vi "chopdata2.vi"(8 "velo":dbl[][](array[numeric]), 9 "pos":dbl[](array[numeric])) -> (1 "slam_pos":dbl[](array[numeric]))   [LabVIEW 2012]
uses:
  G_SEN.vi
  <vilib>/Analysis/baseanly.llb/Real A x B.vi
  <vilib>/Analysis/7linalg.llb/Real SVD Decomposition.vi
  <vilib>/Analysis/Matrix/Numeric/Multiply/Multiply - RM,RM.vi
  <vilib>/Analysis/baseanly.llb/A x Vector.vi
  <vilib>/Analysis/Matrix/Numeric/Conversions/Matrix To Array - RM.vi
  <vilib>/Analysis/NI_AALBase.lvlib
  <vilib>/Analysis/NI_AALPro.lvlib
  <vilib>/Analysis/Matrix/NI_Matrix.lvlib
panel:
  out "Array 2":dbl[][](array[numeric])
  out "Array":dbl[](array[numeric])
  out "thresh":dbl
  out "iter":i32
  in  "y 2":dbl
  in  "graph":bool
  out "error":dbl
  out "R'":dbl[][](array[numeric])
  out "y'":dbl
  out "x'":dbl
  out "mindata":dbl[][](array[numeric])
  out "keydata":dbl[][](array[numeric])
  out "zero_80_240":i32[][](array[numeric])
  out "time":u32
  out "x":dbl[](array[numeric])
  out "y":dbl[](array[numeric])
  out "XY Graph":cluster{"Y":dbl[], "Y":dbl[]}[](graph)
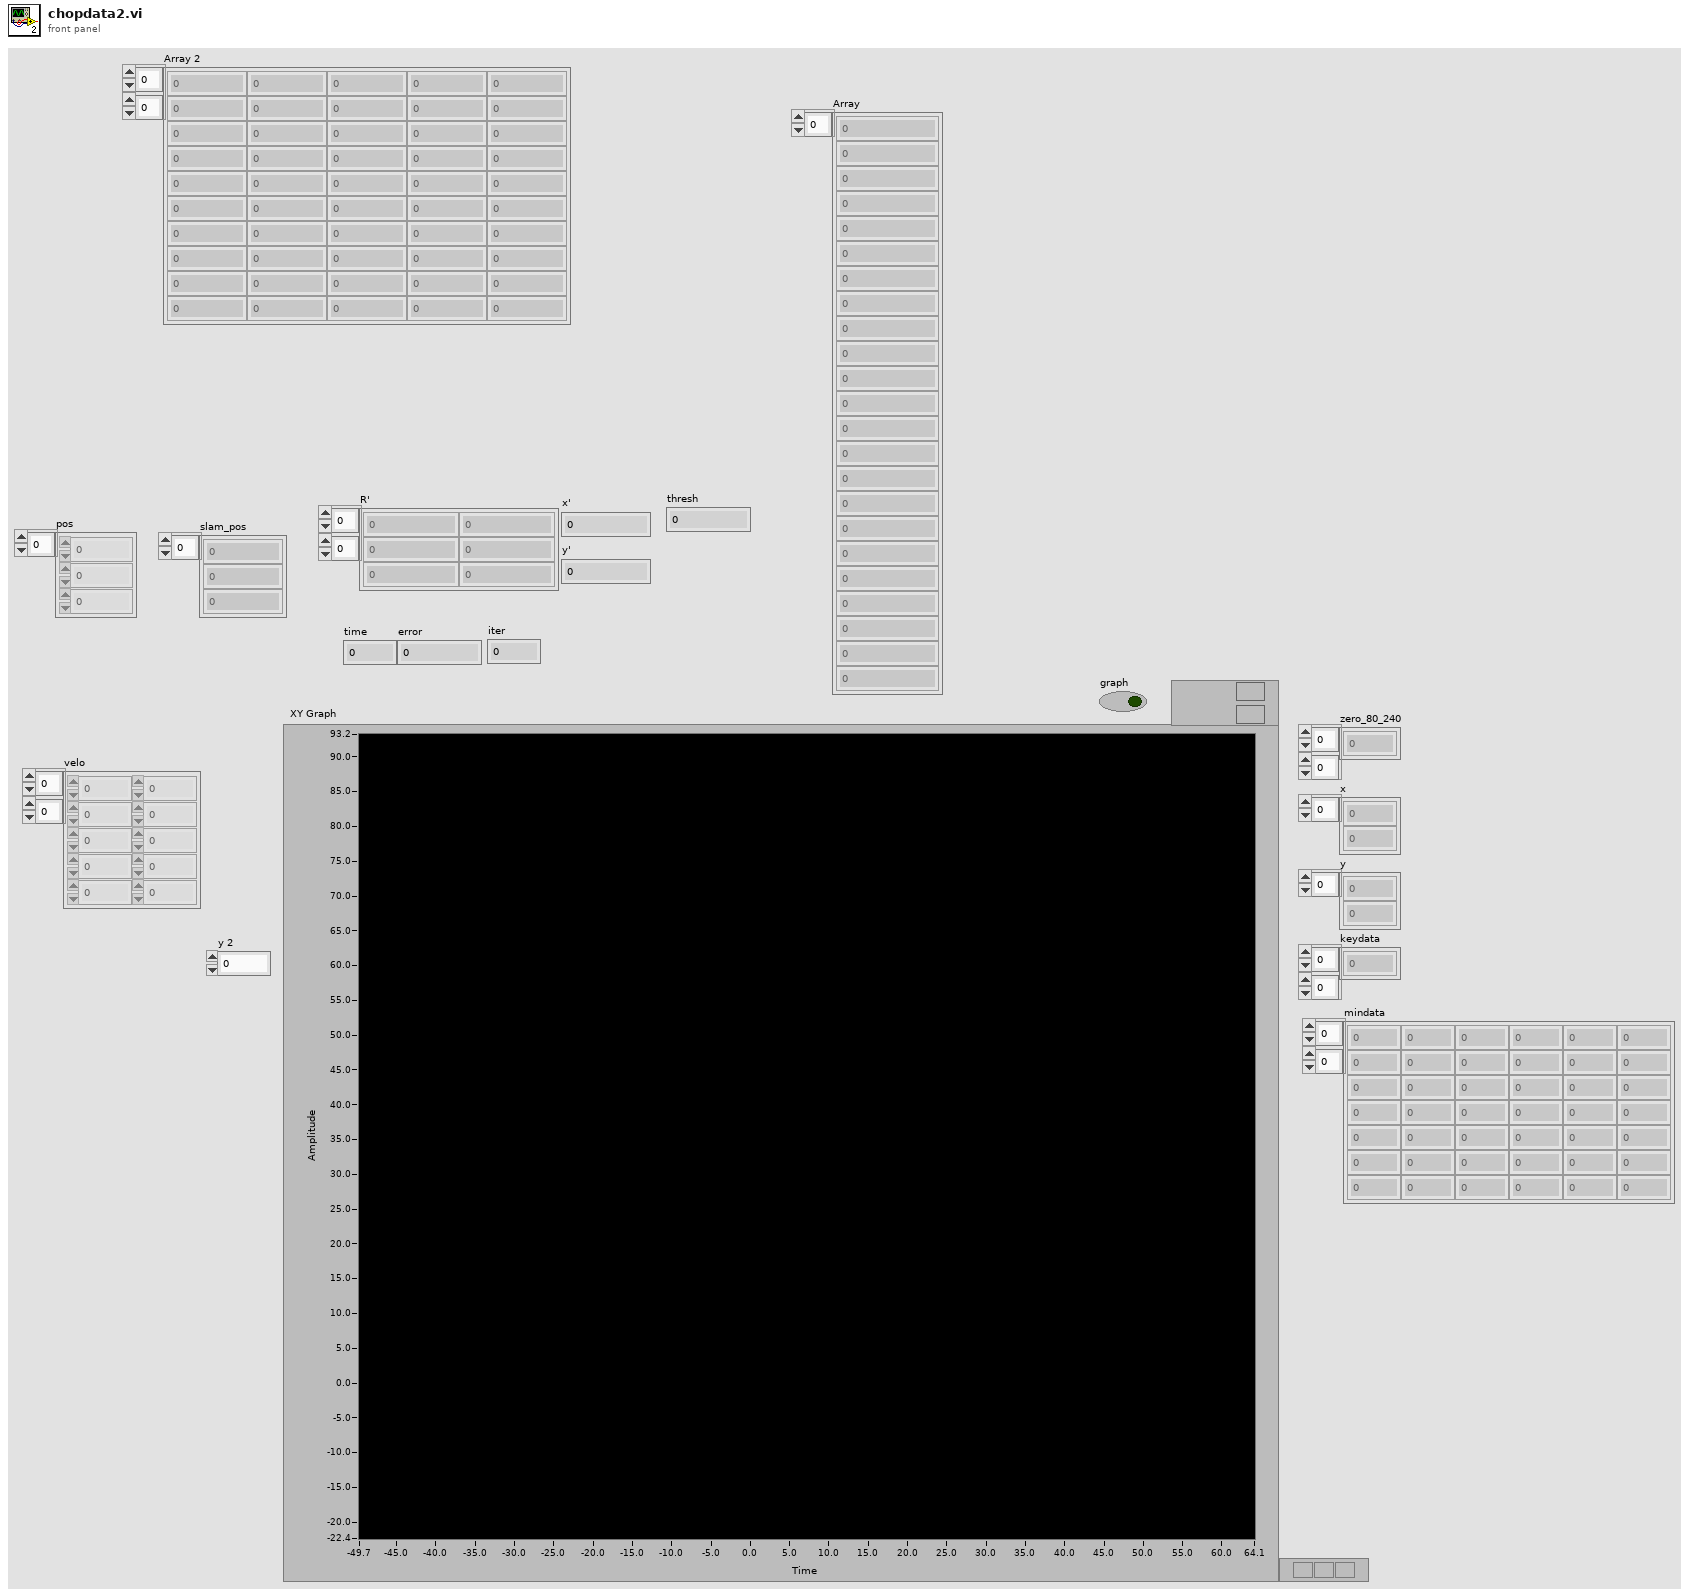
[diagram p1: front panel]
types:
  T1 = cluster{bool, "element":dbl, "element":dbl, "element":dbl}[]
  T2 = cluster{"element":bool, "element":dbl, "element":dbl, "element":dbl}[]
  T3 = typedef "NI_Matrix.lvlib/RealMatrix.ctl" = dbl[][]
  T4 = cluster{"Real Matrix Element":bool, "Real Matrix Element":dbl, "Real Matrix Element":dbl}[]
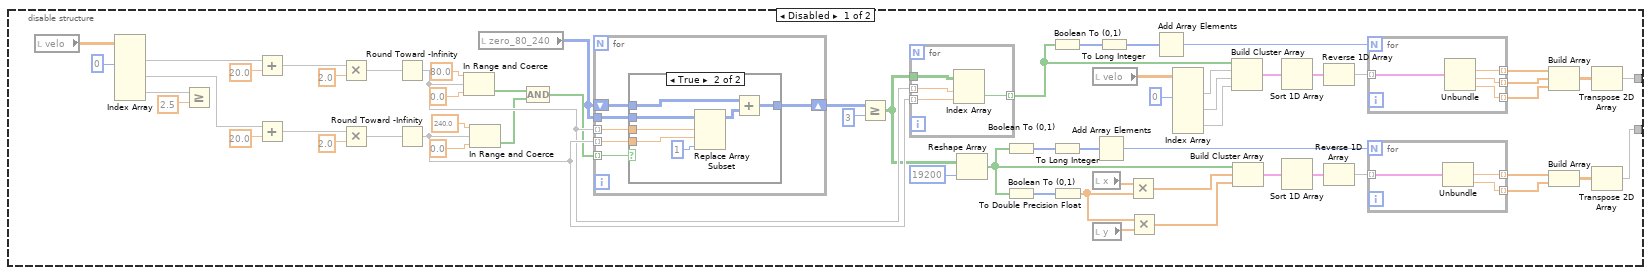
[diagram p3: hidden frame]
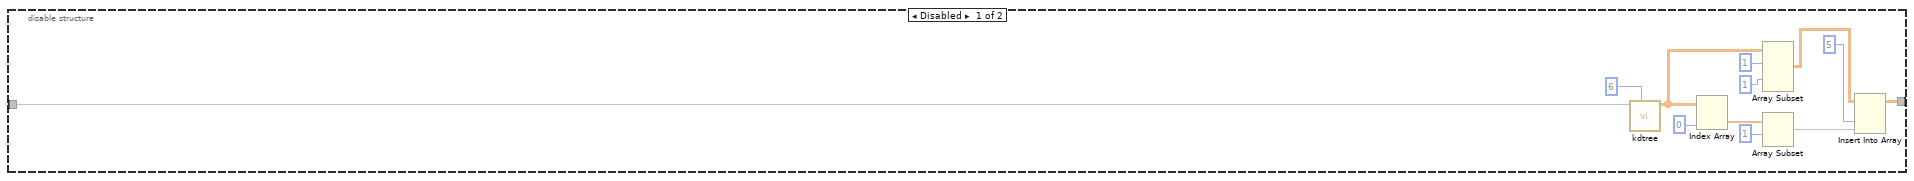
[diagram p5: hidden frame]
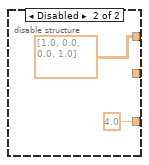
[diagram p7: hidden frame]
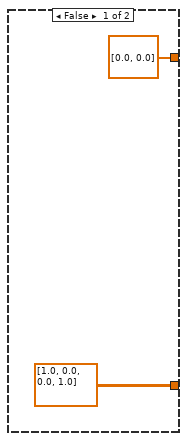
[diagram p9: hidden frame]
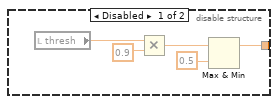
[diagram p10: hidden frame]
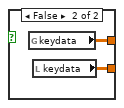
[diagram p12: hidden frame]
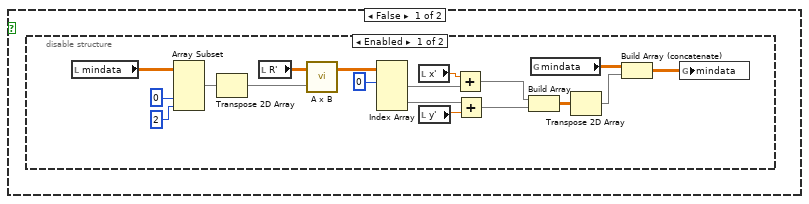
[diagram p13: hidden frame]
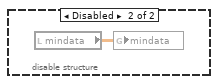
[diagram p15: hidden frame]
diagram:
  n1 = flat-sequence {
    tunnel: [w37] -> w6
    tunnel: w6 -> [w40]
    tunnel: [w40] -> w1
    tunnel: w1 -> [w255]
    tunnel: [w255] -> w5
    tunnel: w5 -> [w265]
    tunnel: [w265] -> w4
    tunnel: w4 -> [w295]
    tunnel: [w295] -> w3
    tunnel: w3 -> [w518]
    tunnel: [w518] -> w2
    tunnel: w2 -> [w520]
    frame #0 {
      n2 = First Call?() -> (First Call?: T/F=w7:bool)
      n3 = case shown="True" w7 {
        frame False {
        }
        frame True {
          n4 = Initialize Array(0, 80 ("dimension size"), 240 ("dimension size")) -> (→"zero_80_240":i32[][])
          n5 = for {
            N: 80 -> [_]
            tunnel: -19.75 -> [w27]
            tunnel: [w24] -> w12 mode=indexing
            tunnel: [w23] -> w17 mode=indexing
            i -> [w26]
            n6 = To Double Precision Float(number=w26) -> (double precision float=w22:dbl)
            n7 = Multiply(x=w22, y=0.5) -> (x*y=w20:dbl)
            n8 = Add(x=w27, y=w20) -> (x+y=w25:dbl)
            n9 = for {
              N: 240 -> [_]
              tunnel: -19.75 -> [w36]
              tunnel: [w34] -> w23 mode=indexing
              tunnel: w25 -> [w33]
              tunnel: [w33] -> w24 mode=indexing
              i -> [w35]
              n10 = To Double Precision Float(number=w35) -> (double precision float=w32:dbl)
              n11 = Multiply(x=w32, y=0.5) -> (x*y=w30:dbl)
              n12 = Add(x=w36, y=w30) -> (x+y=w34:dbl)
            }
          }
          n13 = Reshape Array(w17, 19200 ("dimension size")) -> (→"y":dbl[])
          n14 = Reshape Array(w12, 19200 ("dimension size")) -> (→"x":dbl[])
        }
      }
    }
    frame #1 {
      n15 = Tick Count (ms)() -> (millisecond timer value=w37:u32)
    }
    frame #2 {
      n16 = disable-structure shown="Enabled" {
        disable-tunnel: [w44 w129] -> w39
        disable-tunnel: [w43 w128] -> w38
        frame Disabled {
          n17 = local read "velo"() -> (w50:dbl[][])
          n18 = Index Array(array=w50, index (col) #1=0 ("disabled index (col)")) -> (element #1=w79:dbl[], element #2=w78:dbl[], element #3=w42:dbl[])  [unwired: 5 in]
          n19 = Greater Or Equal?(x=w42, y=2.5) -> ()  [unwired: 1 out]
          n20 = Add(x=w79, y=20.0) -> (x+y=w75:dbl[])
          n21 = Add(x=w78, y=20.0) -> (x+y=w71:dbl[])
          n22 = Multiply(x=w75, y=2.0) -> (x*y=w74:dbl[])
          n23 = Multiply(x=w71, y=2.0) -> (x*y=w70:dbl[])
          n24 = Round Toward -Infinity(1:w74) -> (0:w92:dbl[])
          n25 = Round Toward -Infinity(1:w70) -> (0:w93:dbl[])
          n26 = In Range and Coerce(upper limit=80.0, x=w92, lower limit=0.0) -> (In Range?=w87:bool[])  [unwired: 1 out]
          n27 = In Range and Coerce(upper limit=240.0, x=w93, lower limit=0.0) -> (In Range?=w88:bool[])  [unwired: 1 out]
          n28 = local read "zero_80_240"() -> (w54:i32[][])
          n29 = Compound Arithmetic op=AND(w87, w88) -> (w89:bool[])
          n30 = for {
            shift-right: [w117] -> w91
            shift-left: w54 -> [w118]
            tunnel: w89 -> [w119] mode=indexing
            tunnel: w54 -> [w116]
            tunnel: w92 -> [w115] mode=indexing
            tunnel: w93 -> [w114] mode=indexing
            n31 = case shown="True" w119 {
              tunnel: w118 -> [w120 w123]
              tunnel: [w120 w121] -> w117
              tunnel: w116 -> [_ w127]
              tunnel: w115 -> [_ w126]
              tunnel: w114 -> [_ w125]
              frame False {
              }
              frame True {
                n32 = Replace Array Subset(array=w127, new element=1 ("new element/subarray"), index (row)=w126, index (col)=w125) -> (w122:i32[][])
                n33 = Add(x=w123, y=w122) -> (x+y=w121:i32[][])
              }
            }
          }
          n34 = Greater Or Equal?(x=w91, y=3) -> (x >= y?=w63:bool[][])
          n35 = for {
            tunnel: w63 -> [w113]
            tunnel: w92 -> [w112] mode=indexing
            tunnel: w93 -> [w111] mode=indexing
            tunnel: [w110] -> w96 mode=indexing
            n36 = Index Array(array=w113, index (row)=w112, index (col)=w111) -> (element=w110:bool)
          }
          n37 = Reshape Array(w63, 19200 ("dimension size")) -> (w57:bool[])
          n38 = Boolean To (0,1)(Boolean=w57) -> (0, 1=w59:i16[])
          n39 = Boolean To (0,1)(Boolean=w57) -> (0, 1=w68:i16[])
          n40 = Boolean To (0,1)(Boolean=w96) -> (0, 1=w97:i16[])
          n41 = To Long Integer(number=w59) -> (32bit integer=w58:i32[])
          n42 = To Double Precision Float(number=w68) -> (double precision float=w62:dbl[])
          n43 = local read "velo"() -> (w49:dbl[][])
          n44 = local read "x"() -> (w66:dbl[])
          n45 = local read "y"() -> (w67:dbl[])
          n46 = Add Array Elements(numeric array=w58) -> (sum=w56:i32)
          n47 = To Long Integer(number=w97) -> (32bit integer=w98:i32[])
          n48 = Multiply(x=w66, y=w62) -> (x*y=w65:dbl[])
          n49 = Multiply(x=w62, y=w67) -> (x*y=w64:dbl[])
          n50 = Add Array Elements(numeric array=w98) -> (sum=w99:i32)
          n51 = Index Array(array=w49, index (col) #1=0 ("disabled index (col)")) -> (element #1=w47:dbl[], element #2=w46:dbl[], element #3=w45:dbl[])  [unwired: 5 in]
          n52 = Build Cluster Array(w96, w47, w46, w45) -> (w94:T1)
          n53 = Build Cluster Array(w57, w65, w64) -> (w60:cluster{bool, dbl, dbl}[])
          n54 = Sort 1D Array(array=w94) -> (sorted array=w95:T1)
          n55 = Sort 1D Array(array=w60) -> (sorted array=w61:cluster{bool, dbl, dbl}[])
          n56 = Reverse 1D Array(array=w95) -> (reversed array=w100:T1)
          n57 = Reverse 1D Array(array=w61) -> (reversed array=w55:cluster{bool, dbl, dbl}[])
          n58 = for {
            N: w99 -> [_]
            tunnel: w100 -> [w109] mode=indexing
            tunnel: [w108] -> w77 mode=indexing
            tunnel: [w107] -> w76 mode=indexing
            tunnel: [w106] -> w101 mode=indexing
            n59 = Unbundle(w109) -> ("element"=w108:dbl, "element"=w107:dbl, "element"=w106:dbl)  [unwired: 1 out]
          }
          n60 = for {
            N: w56 -> [_]
            tunnel: w55 -> [w105] mode=indexing
            tunnel: [w104] -> w53 mode=indexing
            tunnel: [w103] -> w52 mode=indexing
            n61 = Unbundle(w105) -> (w104:dbl, w103:dbl)  [unwired: 1 out]
          }
          n62 = Build Array(w77, w76, w101) -> (w102:dbl[][])
          n63 = Build Array(w53, w52) -> (w51:dbl[][])
          n64 = Transpose 2D Array(2D array=w102) -> (transposed array=w44:dbl[][])
          n65 = Transpose 2D Array(2D array=w51) -> (transposed array=w43:dbl[][])
        }
        frame Enabled {
          n66 = local read "velo"() -> (w130:dbl[][])
          n67 = flat-sequence {
            tunnel: w130 -> [w158]
            tunnel: [w133] -> w129
            frame #0 {
              n68 = Index Array(array=w158, index (col) #1=0 ("disabled index (col)")) -> (element #1=w157:dbl[], element #2=w152:dbl[], element #3=w132:dbl[])  [unwired: 5 in]
              n69 = Greater?(x=w132, y=0) -> ()  [unwired: 1 out]
              n70 = In Range and Coerce(upper limit=40.0, x=w152, lower limit=0.0) -> (In Range?=w150:bool[])  [unwired: 1 out]
              n71 = In Range and Coerce(upper limit=40.0, x=w157, lower limit=-40.0) -> (In Range?=w151:bool[])  [unwired: 1 out]
              n72 = local read "velo"() -> (w139:dbl[][])
              n73 = Compound Arithmetic op=AND(w151, w150) -> (w134:bool[])
              n74 = Index Array(array=w139, index (col) #1=0 ("disabled index (col)")) -> (element #1=w137:dbl[], element #2=w136:dbl[], element #3=w135:dbl[])  [unwired: 5 in]
              n75 = Boolean To (0,1)(Boolean=w134) -> (0, 1=w144:i16[])
              n76 = Build Cluster Array(w134, w137, w136, w135) -> (w142:T2)
              n77 = To Long Integer(number=w144) -> (32bit integer=w145:i32[])
              n78 = Sort 1D Array(array=w142) -> (sorted array=w143:T2)
              n79 = Add Array Elements(numeric array=w145) -> (sum=w146:i32)
              n80 = Reverse 1D Array(array=w143) -> (reversed array=w147:T2)
              n81 = for {
                N: w146 -> [_]
                tunnel: w147 -> [w163] mode=indexing
                tunnel: [w162] -> w141 mode=indexing
                tunnel: [w161] -> w140 mode=indexing
                tunnel: [w160] -> w148 mode=indexing
                n82 = Unbundle(w163) -> ("element"=w162:dbl, "element"=w161:dbl, "element"=w160:dbl)  [unwired: 1 out]
              }
              n83 = Build Array(w141, w140, w148) -> (w149:dbl[][])
              n84 = Transpose 2D Array(2D array=w149) -> (transposed array=w133:dbl[][])
            }
          }
          n85 = disable-structure shown="Enabled" {
            disable-tunnel: w129 -> [w175 w183]
            disable-tunnel: [w167 w176] -> w128
            frame Disabled {
              n86 = call "kdtree.vi"("depth_max"=6, "in"=w175) -> ("out"=w171:dbl[][])  [unwired: 8 in, 1 out]
              n87 = Index Array(array=w171, index (col)=0 ("disabled index (col)")) -> (element=w166:dbl[])  [unwired: 1 in]
              n88 = Array Subset(array=w171, index (row)=1 ("index"), index (col)=1 ("index")) -> (w169:dbl[][])  [unwired: 2 in]
              n89 = Array Subset(array=w166, index=1) -> (w164:dbl[])  [unwired: 1 in]
              n90 = Insert Into Array(array=w169, index (col)=5 ("disabled index (col)"), new element=w164) -> (w167:dbl[][])  [unwired: 1 in]
            }
            frame Enabled {
              n91 = Index Array(array=w183, index (col) #1=0 ("disabled index (col)"), index (col) #2=0 ("index (col)"), index (col) #3=1 ("index (col)"), index (col) #4=1 ("index (col)")) -> (element #1=w185:dbl[], element #2=w188:dbl[], element #3=w187:dbl[], element #4=w186:dbl[])  [unwired: 4 in]
              n92 = for {
                tunnel: w188 -> [w252] mode=indexing
                tunnel: w187 -> [w251]
                tunnel: w186 -> [w250] mode=indexing
                tunnel: w185 -> [w249]
                tunnel: [w239] -> w184 mode=indexing
                n93 = Subtract(x=w249, y=w252) -> (x-y=w248:dbl[])
                n94 = Subtract(x=w251, y=w250) -> (x-y=w247:dbl[])
                n95 = Square(x=w248) -> (x^2=w246:dbl[])
                n96 = Square(x=w247) -> (x^2=w245:dbl[])
                n97 = Add(x=w246, y=w245) -> (x+y=w244:dbl[])
                n98 = Less Or Equal?(x=w244, y=1.0) -> (x <= y?=w242:bool[])
                n99 = Boolean To (0,1)(Boolean=w242) -> (0, 1=w241:i16[])
                n100 = To Long Integer(number=w241) -> (32bit integer=w240:i32[])
                n101 = Add Array Elements(numeric array=w240) -> (sum=w239:i32)
              }
              n102 = Index Array(array=w183, index (col) #1=0 ("disabled index (col)")) -> (element #1=w182:dbl[], element #2=w180:dbl[])  [unwired: 3 in]
              n103 = while {
                shift-right: [w200] -> _
                shift-left: w184 -> [w196]
                tunnel: w182 -> [w208]
                tunnel: w180 -> [w207]
                tunnel: [w209] -> w179 mode=indexing
                tunnel: [w206] -> w178 mode=indexing
                stop <- w197 stop-if-true
                n104 = Array Max & Min(array=w196) -> (max value=w199:i32, max index (indices)=w195:i32)  [unwired: 2 out]
                n105 = Index Array(array=w208, index=w195) -> (element=w238:dbl)
                n106 = Index Array(array=w207, index=w195) -> (element=w237:dbl)
                n107 = Greater?(x=3, y=w199) -> (0:w197:bool)
                n108 = Replace Array Subset(array=w196, new element=0 ("new element/subarray"), index=w195) -> (w193:i32[])
                n109 = Subtract(x=w208, y=w238) -> (x-y=w232:dbl[])
                n110 = Subtract(x=w207, y=w237) -> (x-y=w231:dbl[])
                n111 = Square(x=w232) -> (x^2=w233:dbl[])
                n112 = Square(x=w231) -> (x^2=w234:dbl[])
                n113 = Add(x=w233, y=w234) -> (x+y=w235:dbl[])
                n114 = Less Or Equal?(x=w235, y=1.0) -> (x <= y?=w230:bool[])
                n115 = Boolean To (0,1)(Boolean=w230) -> (0, 1=w229:i16[])
                n116 = To Double Precision Float(number=w229) -> (double precision float=w222:dbl[])
                n117 = Multiply(x=w208, y=w222) -> (x*y=w228:dbl[])
                n118 = Add Array Elements(numeric array=w222) -> (sum=w226:dbl)
                n119 = Multiply(x=w207, y=w222) -> (x*y=w223:dbl[])
                n120 = Add Array Elements(numeric array=w222) -> (sum=w225:dbl)
                n121 = Add Array Elements(numeric array=w228) -> (sum=w227:dbl)
                n122 = Add Array Elements(numeric array=w223) -> (sum=w224:dbl)
                n123 = Divide(x=w227, y=w226) -> (x/y=w221:dbl)
                n124 = Divide(x=w224, y=w225) -> (x/y=w220:dbl)
                n125 = Subtract(x=w208, y=w221) -> (x-y=w217:dbl[])
                n126 = Subtract(x=w207, y=w220) -> (x-y=w216:dbl[])
                n127 = Square(x=w217) -> (x^2=w219:dbl[])
                n128 = Square(x=w216) -> (x^2=w218:dbl[])
                n129 = Add(x=w219, y=w218) -> (x+y=w215:dbl[])
                n130 = Array Max & Min(array=w215) -> (min index (indices)=w214:i32)  [unwired: 3 out]
                n131 = Index Array(array=w208, index=w214) -> (element=w209:dbl)
                n132 = Index Array(array=w207, index=w214) -> (element=w206:dbl)
                n133 = Subtract(x=w208, y=w209) -> (x-y=w212:dbl[])
                n134 = Subtract(x=w207, y=w206) -> (x-y=w213:dbl[])
                n135 = Square(x=w212) -> (x^2=w210:dbl[])
                n136 = Square(x=w213) -> (x^2=w211:dbl[])
                n137 = Add(x=w210, y=w211) -> (x+y=w205:dbl[])
                n138 = Greater?(x=w205, y=1.0) -> (0:w203:bool[])
                n139 = Boolean To (0,1)(Boolean=w203) -> (0, 1=w202:i16[])
                n140 = To Long Integer(number=w202) -> (32bit integer=w201:i32[])
                n141 = Multiply(x=w201, y=w193) -> (x*y=w200:i32[])
              }
              n142 = Build Array(w179, w178) -> (w177:dbl[][])
              n143 = Transpose 2D Array(2D array=w177) -> (transposed array=w176:dbl[][])
            }
          }
        }
      }
      "keydata" <- w39
      "mindata" <- w38
    }
    frame #3 {
      n144 = global read "G_SEN.vi" "keydata"() -> (w253:dbl[][])
      n145 = Empty Array?(array=w253) -> (empty?=w254:bool)
      n146 = case shown="True" w254 {
        frame False {
        }
        frame True {
          n147 = local read "pos"() -> (w259:dbl[])
          n148 = local read "mindata"() -> (w258:dbl[][])
          n149 = local read "keydata"() -> (w257:dbl[][])
          n150 = global write "G_SEN.vi" "pos_velo_key"(w259) -> ()
          n151 = global write "G_SEN.vi" "keydata"(w257) -> ()
          n152 = global write "G_SEN.vi" "mindata"(w258) -> ()
          n153 = global write "G_SEN.vi" "pos_slam"(dbl[][] [[1.0, 0.0, 0.0], [0.0, 1.0, 0.0], [0.0, 0.0, 1.0]]) -> ()
        }
      }
    }
    frame #4 {
      n154 = disable-structure shown="Enabled" {
        disable-tunnel: [w278 _] -> w264
        disable-tunnel: [w277 4.0 ("y'")] -> w263
        disable-tunnel: [w267 dbl[][] [[1.0, 0.0], [0.0, 1.0]]] -> w261
        frame Enabled {
          n155 = global read "G_SEN.vi" "pos_velo_key"() -> (w275:dbl[])
          n156 = local read "pos"() -> (w276:dbl[])
          n157 = Subtract(x=w276, y=w275) -> (x-y=w274:dbl[])
          n158 = global read "G_SEN.vi" "pos_velo_key"() -> (w288:dbl[])
          n159 = Index Array(array=w274, index=2) -> (element=w266:dbl)
          n160 = Sine & Cosine(0:w266) -> (1:w272:dbl, 2:w270:dbl)
          n161 = Negate(x=w272) -> (-x=w271:dbl)
          n162 = Build Array(w270, w272) -> (w269:dbl[])
          n163 = local read "pos"() -> (w282:dbl[])
          n164 = Index Array(array=w288, index #1=0 ("index")) -> (element #1=w286:dbl, element #2=w285:dbl, element #3=w284:dbl)  [unwired: 2 in]
          n165 = Build Array(w271, w270) -> (w268:dbl[])
          n166 = Negate(x=w284) -> (-x=w283:dbl)
          n167 = Index Array(array=w282, index #1=0 ("index")) -> (element #1=w280:dbl, element #2=w279:dbl)  [unwired: 1 in]
          n168 = Build Array(w269, w268) -> (w267:dbl[][])
          n169 = call "rotm_siso.vi"("angle[rad]"=w283, "y0"=w285, "x0"=w286, "y"=w279, "x"=w280) -> ("y'"=w277:dbl, "x'"=w278:dbl)  [unwired: 5 in]
        }
        frame Disabled {
        }
      }
      "x'" <- w264
      "y'" <- w263
      "R'" <- w261
      "error" <- inf
      "thresh" <- 3.0 ("thresh")
    }
    frame #5 {
      n170 = for {
        N: 20 -> [_]
        tunnel: [w298] -> w293
        tunnel: [w297] -> w292 mode=indexing
        tunnel: [w296] -> w291 mode=indexing
        i -> [w298]
        stop <- w299 continue-if-true
        n171 = disable-structure shown="Enabled" {
          disable-tunnel: [w317 _] -> w299
          disable-tunnel: [w308 _] -> w297
          disable-tunnel: [w306 _] -> w296
          frame Enabled {
            (unwired) cluster{"Y":dbl[], "Y":dbl[]}[] [{"Y"=array[263 elements], "Y"=array[263 elements]}, {"Y"=array[263 elements], "Y"=array[263 elements]}] ("XY Graph 2")
            n172 = local read "mindata"() -> (w352:dbl[][])
            n173 = Array Subset(array=w352, index (col)=0 ("index"), length (col)=2 ("length")) -> (w349:dbl[][])  [unwired: 2 in]
            n174 = Transpose 2D Array(2D array=w349) -> (transposed array=w346:dbl[][])
            n175 = local read "R'"() -> (w347:dbl[][])
            n176 = call-poly <vilib>:"A x B.vi"("B"=w346, "A"=w347) -> ("A x B"=w345:T3)  [unwired: 1 out]
            n177 = Index Array(array=w345, index (row) #1=0 ("index (row)")) -> (element #1=w344:dbl[], element #2=w337:dbl[])  [unwired: 3 in]
            n178 = global read "G_SEN.vi" "mindata"() -> (w338:dbl[][])
            n179 = local read "x'"() -> (w354:dbl)
            n180 = local read "y'"() -> (w353:dbl)
            n181 = Add(x=w354, y=w344) -> (x+y=w343:dbl[])
            n182 = Add(x=w337, y=w353) -> (x+y=w342:dbl[])
            n183 = Index Array(array=w338, index (col) #1=0 ("disabled index (col)")) -> (element #1=w340:dbl[], element #2=w339:dbl[])  [unwired: 3 in]
            n184 = for {
              tunnel: w343 -> [w478] mode=indexing
              tunnel: w342 -> [w477] mode=indexing
              tunnel: w340 -> [w479]
              tunnel: w339 -> [w474]
              tunnel: [w478] -> w334 mode=indexing
              tunnel: [w477] -> w333 mode=indexing
              tunnel: [w476] -> w336 mode=indexing
              tunnel: [w473] -> w335 mode=indexing
              tunnel: [w471] -> w331 mode=indexing
              n185 = Subtract(x=w479, y=w478) -> (x-y=w484:dbl[])
              n186 = Subtract(x=w474, y=w477) -> (x-y=w483:dbl[])
              n187 = Square(x=w484) -> (x^2=w482:dbl[])
              n188 = Square(x=w483) -> (x^2=w481:dbl[])
              n189 = Add(x=w482, y=w481) -> (x+y=w480:dbl[])
              n190 = Array Max & Min(array=w480) -> (min value=w472:dbl, min index (indices)=w475:i32)  [unwired: 2 out]
              n191 = Square Root(x=w472) -> (sqrt(x)=w471:dbl)
              n192 = Index Array(array=w479, index=w475) -> (element=w476:dbl)
              n193 = Index Array(array=w474, index=w475) -> (element=w473:dbl)
            }
            n194 = local read "thresh"() -> (w307:dbl)
            n195 = Build Cluster Array(w331, w336, w335, w334, w333) -> (w332:cluster{dbl, dbl, dbl, dbl, dbl}[])
            n196 = Greater?(x=w307, y=w331) -> (0:w330:bool[])
            n197 = Sort 1D Array(array=w332) -> (sorted array=w327:cluster{dbl, dbl, dbl, dbl, dbl}[])
            n198 = Boolean To (0,1)(Boolean=w330) -> (0, 1=w329:i16[])
            n199 = To Long Integer(number=w329) -> (32bit integer=w328:i32[])
            n200 = Add Array Elements(numeric array=w328) -> (sum=w319:i32)
            n201 = for {
              N: w319 -> [_]
              tunnel: w327 -> [w470] mode=indexing
              tunnel: [w469] -> w324 mode=indexing
              tunnel: [w468] -> w323 mode=indexing
              tunnel: [w467] -> w325 mode=indexing
              tunnel: [w466] -> w326 mode=indexing
              tunnel: [w465] -> w322 mode=indexing
              n202 = Unbundle(w470) -> (w465:dbl, w469:dbl, w468:dbl, w467:dbl, w466:dbl)
            }
            n203 = Less Or Equal?(x=3, y=w319) -> (x <= y?=w316:bool)
            n204 = Add Array Elements(numeric array=w322) -> (sum=w321:dbl)
            n205 = Divide(x=w321, y=w319) -> (x/y=w309:dbl)
            n206 = local read "error"() -> (w311:dbl)
            n207 = local read "error"() -> (w315:dbl)
            n208 = Subtract(x=w309, y=w315) -> (x-y=w314:dbl)
            n209 = Max & Min(x=w311, y=w309) -> (min(x,y)=w310:dbl)  [unwired: 1 out]
            n210 = local write "error"(w310) -> ()
            n211 = Less?(x=w314, y=-0.0001) -> (x < y?=w312:bool)
            n212 = And(x=w312, y=w316) -> (x .and. y?=w317:bool)
            n213 = case shown="True" w317 {
              tunnel: [dbl[][] [[1.0, 0.0], [0.0, 1.0]] w424] -> w320
              tunnel: w324 -> [_ w422]
              tunnel: w323 -> [_ w421]
              tunnel: w326 -> [_ w420]
              tunnel: w325 -> [_ w419]
              tunnel: [dbl[] [0.0, 0.0] w414] -> w303
              frame False {
              }
              frame True {
                n214 = disable-structure shown="Enabled" {
                  disable-tunnel: [w431 w433] -> w411
                  frame Disabled {
                    n215 = local read "thresh"() -> (w429:dbl)
                    n216 = Multiply(x=w429, y=0.9) -> (x*y=w432:dbl)
                    n217 = Max & Min(x=w432, y=0.5) -> (max(x,y)=w431:dbl)  [unwired: 1 out]
                  }
                  frame Enabled {
                    n218 = local read "thresh"() -> (w438:dbl)
                    n219 = local read "error"() -> (w439:dbl)
                    n220 = Add(x=w439, y=w438) -> (x+y=w437:dbl)
                    n221 = Multiply(x=w437, y=0.5) -> (x*y=w435:dbl)
                    n222 = Max & Min(x=w435, y=0.2) -> (max(x,y)=w433:dbl)  [unwired: 1 out]
                  }
                }
                n223 = flat-sequence {
                  tunnel: w422 -> [w451]
                  tunnel: w421 -> [w450]
                  tunnel: [w447] -> w415
                  tunnel: [w446] -> w413
                  frame #0 {
                    n224 = Add Array Elements(numeric array=w451) -> (sum=w445:dbl)
                    n225 = Add Array Elements(numeric array=w450) -> (sum=w441:dbl)
                    n226 = Array Size(array=w451) -> (size(s)=w444:i32)
                    n227 = Array Size(array=w450) -> (size(s)=w442:i32)
                    n228 = Divide(x=w445, y=w444) -> (x/y=w449:dbl)
                    n229 = Divide(x=w441, y=w442) -> (x/y=w448:dbl)
                    n230 = Subtract(x=w451, y=w449) -> (x-y=w443:dbl[])
                    n231 = Subtract(x=w450, y=w448) -> (x-y=w440:dbl[])
                    n232 = Build Array(w449, w448) -> (w447:dbl[])
                    n233 = Build Array(w443, w440) -> (w446:dbl[][])
                  }
                }
                n234 = flat-sequence {
                  tunnel: w420 -> [w464]
                  tunnel: w419 -> [w463]
                  tunnel: [w460] -> w417
                  tunnel: [w459] -> w412
                  frame #0 {
                    n235 = Add Array Elements(numeric array=w463) -> (sum=w454:dbl)
                    n236 = Add Array Elements(numeric array=w464) -> (sum=w458:dbl)
                    n237 = Array Size(array=w463) -> (size(s)=w455:i32)
                    n238 = Array Size(array=w464) -> (size(s)=w457:i32)
                    n239 = Divide(x=w454, y=w455) -> (x/y=w462:dbl)
                    n240 = Divide(x=w458, y=w457) -> (x/y=w461:dbl)
                    n241 = Subtract(x=w463, y=w462) -> (x-y=w453:dbl[])
                    n242 = Subtract(x=w464, y=w461) -> (x-y=w456:dbl[])
                    n243 = Build Array(w462, w461) -> (w460:dbl[])
                    n244 = Build Array(w453, w456) -> (w452:dbl[][])
                    n245 = Transpose 2D Array(2D array=w452) -> (transposed array=w459:dbl[][])
                  }
                }
                n246 = local write "thresh"(w411) -> ()
                n247 = call-poly <vilib>:"A x B.vi"("B"=w412, "A"=w413) -> ("A x B"=w423:T3)  [unwired: 1 out]
                n248 = call-poly <vilib>:"SVD Decomposition.vi"("A"=w423) -> ("Matrix V"=w425:T3, "Matrix U"=w426:T3)  [unwired: 6 in, 3 out]
                n249 = Transpose 2D Array(2D array=w425) -> (transposed array=w427:T3)
                n250 = call-poly <vilib>:"Multiply.vi"("Real Matrix B"=w427, "Real Matrix A"=w426) -> ("A * B"=w418:T3)
                n251 = call-poly <vilib>:"A x B.vi"("Vector"=w417, "A"=w418) -> ("A x Vector"=w416:dbl[])  [unwired: 1 out]
                n252 = call-poly <vilib>:"Matrix To Array.vi"("Real Matrix"=w418) -> ("Real 2D Array"=w424:dbl[][])
                n253 = Subtract(x=w415, y=w416) -> (x-y=w414:dbl[])
              }
            }
            n254 = Square(x=w303) -> (x^2=w305:dbl[])
            n255 = Add Array Elements(numeric array=w305) -> (sum=w304:dbl)
            n256 = Square Root(x=w304) -> (sqrt(x)=w301:dbl)
            n257 = local read "thresh"() -> (w302:dbl)
            n258 = Greater?(x=w302, y=w301) -> (0:w300:bool)
            n259 = case shown="True" w300 {
              tunnel: w320 -> [_ w358]
              tunnel: [_ w357] -> w308
              tunnel: [_ w356] -> w306
              tunnel: w303 -> [_ w355]
              frame False {
              }
              frame True {
                n260 = flat-sequence {
                  tunnel: w355 -> [w359]
                  tunnel: w358 -> [w366]
                  tunnel: [w361] -> w357
                  tunnel: [w359] -> w356
                  frame #0 {
                    n261 = flat-sequence {
                      tunnel: w366 -> [w403]
                      tunnel: [w394] -> w365
                      frame #0 {
                        w408 = 0 ("disabled index (col)")
                        n262 = Index Array(array=w403, index (row) #1=0 ("disabled index (row)"), index (col) #1=1 ("disabled index (col)"), index (row) #2=w408, index (col) #2=w408) -> (element #1=w404:dbl, element #2=w405:dbl)
                        n263 = Inverse Tangent (2 Input)(1:w405, 2:w404) -> (0:w402:dbl)
                        n264 = Multiply(x=w402, y=0.1) -> (x*y=w395:dbl)
                        n265 = Sine & Cosine(0:w395) -> (1:w400:dbl, 2:w398:dbl)
                        n266 = Negate(x=w400) -> (-x=w399:dbl)
                        n267 = Build Array(w398, w400) -> (w397:dbl[])
                        n268 = Build Array(w399, w398) -> (w396:dbl[])
                        n269 = Build Array(w397, w396) -> (w394:dbl[][])
                      }
                    }
                    n270 = local read "x'"() -> (w383:dbl)
                    n271 = local read "y'"() -> (w384:dbl)
                    n272 = Build Array(w383, w384) -> (w382:dbl[])
                    n273 = Multiply(x=dbl[] [0.1, 1.0], y=w359) -> (x*y=w364:dbl[])
                    n274 = local read "R'"() -> (w386:dbl[][])
                    n275 = Insert Into Array(array=w386, index (col)=2 ("disabled index (col)"), new element=w382) -> (w387:dbl[][])  [unwired: 1 in]
                    n276 = Square(x=w364) -> (x^2=w363:dbl[])
                    n277 = Insert Into Array(array=w365, index (col)=2 ("disabled index (col)"), new element=w364) -> (w392:dbl[][])  [unwired: 1 in]
                    n278 = Add Array Elements(numeric array=w363) -> (sum=w362:dbl)
                    n279 = Insert Into Array(array=w392, index (row)=2, new element=dbl[] [0.0, 0.0, 1.0]) -> (w381:dbl[][])  [unwired: 1 in]
                    n280 = Insert Into Array(array=w387, index (row)=2, new element=dbl[] [0.0, 0.0, 1.0]) -> (w380:dbl[][])  [unwired: 1 in]
                    n281 = Square Root(x=w362) -> (sqrt(x)=w361:dbl)
                    n282 = call-poly <vilib>:"A x B.vi"("B"=w380, "A"=w381) -> ("A x B"=w375:T3)  [unwired: 1 out]
                    n283 = call-poly <vilib>:"Matrix To Array.vi"("Real Matrix"=w375) -> ("Real 2D Array"=w373:dbl[][])
                    n284 = Array Subset(array=w373, index (row)=0 ("index"), length (row)=2 ("length"), index (col)=0 ("index"), length (col)=2 ("length")) -> (w374:dbl[][])
                    n285 = Index Array(array=w373, index (row) #1=0 ("disabled index (row)"), index (col) #1=2 ("disabled index (col)"), index (row) #2=1 ("index (row)"), index (col) #2=2 ("disabled index (col)")) -> (element #1=w368:dbl, element #2=w367:dbl)
                    n286 = local write "R'"(w374) -> ()
                    n287 = local write "x'"(w368) -> ()
                    n288 = local write "y'"(w367) -> ()
                  }
                }
              }
            }
          }
          frame Disabled {
          }
        }
      }
      "iter" <- w293
      "Array" <- w292
      "Array 2" <- w291
    }
    frame #6 {
      w488 = 0.0 ("element")
      w513 = 0 ("disabled index (col)")
      n289 = local read "R'"() -> (w495:dbl[][])
      n290 = local read "x'"() -> (w497:dbl)
      n291 = local read "y'"() -> (w496:dbl)
      n292 = global read "G_SEN.vi" "pos_velo_key"() -> (w511:dbl[])
      n293 = Build Array(w497, w496) -> (w493:dbl[])
      n294 = Transpose 2D Array(2D array=w495) -> (transposed array=w494:dbl[][])
      n295 = local read "R'"() -> (w512:dbl[][])
      n296 = Build Array (concatenate)(w494, w493) -> (w492:dbl[][])
      n297 = Index Array(array=w512, index (row) #1=0 ("disabled index (row)"), index (col) #1=1 ("disabled index (col)"), index (row) #2=w513, index (col) #2=w513) -> (element #1=w517:dbl, element #2=w516:dbl)
      n298 = Inverse Tangent (2 Input)(1:w516, 2:w517) -> (0:w498:dbl)
      n299 = Transpose 2D Array(2D array=w492) -> (transposed array=w491:dbl[][])
      n300 = Index Array(array=w511, index #1=0 ("index")) -> (element #1=w509:dbl, element #2=w508:dbl, element #3=w499:dbl)  [unwired: 2 in]
      n301 = Add(x=w499, y=w498) -> (x+y=w501:dbl)
      n302 = Negate(x=w499) -> (-x=w507:dbl)
      n303 = Build Array(w488, w488, 1.0 ("element")) -> (w490:dbl[])
      n304 = global read "G_SEN.vi" "pos_slam"() -> (w486:dbl[][])
      n305 = Build Array (concatenate)(w491, w490) -> (w487:dbl[][])
      n306 = local read "y'"() -> (w505:dbl)
      n307 = local read "x'"() -> (w506:dbl)
      n308 = call-poly <vilib>:"A x B.vi"("B"=w486, "A"=w487) -> ("A x B"=w485:T3)  [unwired: 1 out]
      n309 = call "rotm_siso.vi"("angle[rad]"=w507, "reverse"=TRUE, "y0"=w508, "x0"=w509, "y"=w505, "x"=w506) -> ("y'"=w502:dbl, "x'"=w503:dbl)  [unwired: 4 in]
      n310 = global write "G_SEN.vi" "pos_slam"(w485) -> ()
      n311 = Build Array(w503, w502, w501) -> (→"slam_pos":dbl[])
    }
    frame #7 {
      n312 = Tick Count (ms)() -> (millisecond timer value=w521:u32)
      n313 = Subtract(x=w521, y=w520) -> (x-y=→"time":u32)
    }
    frame #8 {
      n314 = case shown="True" "graph" {
        tunnel: [w551 w553] -> w523
        tunnel: [w550 w552] -> w540
        frame True {
          n315 = global read "G_SEN.vi" "mindata"() -> (w551:dbl[][])
          n316 = local read "mindata"() -> (w550:dbl[][])
        }
        frame False {
          n317 = global read "G_SEN.vi" "keydata"() -> (w553:dbl[][])
          n318 = local read "keydata"() -> (w552:dbl[][])
        }
      }
      n319 = Array Subset(array=w540, index (col)=0 ("index"), length (col)=2 ("length")) -> (w537:dbl[][])  [unwired: 2 in]
      n320 = Transpose 2D Array(2D array=w537) -> (transposed array=w536:dbl[][])
      n321 = local read "R'"() -> (w541:dbl[][])
      n322 = call-poly <vilib>:"A x B.vi"("B"=w536, "A"=w541) -> ("A x B"=w535:T3)  [unwired: 1 out]
      n323 = local read "y'"() -> (w526:dbl)
      n324 = Add(x=w526, y="y 2") -> (x+y=w525:dbl)
      n325 = Index Array(array=w535, index (row) #1=0 ("index (row)")) -> (element #1=w545:dbl[], element #2=w544:dbl[])  [unwired: 3 in]
      n326 = local read "x'"() -> (w546:dbl)
      n327 = Add(x=w544, y=w525) -> (x+y=w542:dbl[])
      n328 = Index Array(array=w523, index (col) #1=0 ("disabled index (col)")) -> (element #1=w522:dbl[], element #2=w548:dbl[])  [unwired: 3 in]
      n329 = Add(x=w546, y=w545) -> (x+y=w543:dbl[])
      n330 = call "Convert to Dynamic Data8"("Array"=w522) -> ("Dynamic Data Type"=w533:dynamicdata)  [unwired: 3 in]
      n331 = call "Convert to Dynamic Data7"("Array"=w548) -> ("Dynamic Data Type"=w530:dynamicdata)  [unwired: 3 in]
      n332 = call "Convert to Dynamic Data12"("Array"=w542) -> ("Dynamic Data Type"=w528:dynamicdata)  [unwired: 3 in]
      n333 = call "Convert to Dynamic Data11"("Array"=w543) -> ("Dynamic Data Type"=w531:dynamicdata)  [unwired: 3 in]
      n334 = Merge Signals(w530, w528) -> (w529:dynamicdata)
      n335 = Merge Signals(w533, w531) -> (w532:dynamicdata)
      n336 = call "Build XY Graph"("Y Input"=w529, "X Input"=w532) -> ("XY Graph"=→"XY Graph":cluster{"Y":dbl[], "Y":dbl[]}[])  [unwired: 3 in, 6 out]
    }
    frame #9 {
      n337 = global read "G_SEN.vi" "pos_velo_key"() -> (w555:dbl[])
      n338 = local read "pos"() -> (w554:dbl[])
      n339 = Subtract(x=w554, y=w555) -> (x-y=w556:dbl[])
      n340 = Square(x=w556) -> (x^2=w557:dbl[])
      n341 = Index Array(array=w557, index #1=0 ("index")) -> (element #1=w559:dbl, element #2=w560:dbl)  [unwired: 1 in]
      n342 = Add(x=w559, y=w560) -> (x+y=w561:dbl)
      n343 = Greater Or Equal?(x=w561, y=50.0) -> (x >= y?=w563:bool)
      n344 = case shown="True" w563 {
        frame False {
          n345 = disable-structure shown="Enabled" {
            frame Enabled {
              n346 = local read "mindata"() -> (w571:dbl[][])
              n347 = Array Subset(array=w571, index (col)=0 ("index"), length (col)=2 ("length")) -> (w578:dbl[][])  [unwired: 2 in]
              n348 = Transpose 2D Array(2D array=w578) -> (transposed array=w579:dbl[][])
              n349 = local read "R'"() -> (w575:dbl[][])
              n350 = call-poly <vilib>:"A x B.vi"("B"=w579, "A"=w575) -> ("A x B"=w580:T3)  [unwired: 1 out]
              n351 = Index Array(array=w580, index (row) #1=0 ("index (row)")) -> (element #1=w573:dbl[], element #2=w574:dbl[])  [unwired: 3 in]
              n352 = local read "x'"() -> (w572:dbl)
              n353 = local read "y'"() -> (w570:dbl)
              n354 = Add(x=w572, y=w573) -> (x+y=w569:dbl[])
              n355 = Add(x=w574, y=w570) -> (x+y=w568:dbl[])
              n356 = Build Array(w569, w568) -> (w567:dbl[][])
              n357 = global read "G_SEN.vi" "mindata"() -> (w566:dbl[][])
              n358 = Transpose 2D Array(2D array=w567) -> (transposed array=w564:dbl[][])
              n359 = Build Array (concatenate)(w566, w564) -> (w565:dbl[][])
              n360 = global write "G_SEN.vi" "mindata"(w565) -> ()
            }
            frame Disabled {
            }
          }
        }
        frame True {
          n361 = local read "slam_pos"() -> (w583:dbl[])
          n362 = disable-structure shown="Enabled" {
            frame Enabled {
              n363 = global read "G_SEN.vi" "mindata"() -> (w597:dbl[][])
              n364 = Index Array(array=w597, index (col) #1=0 ("disabled index (col)")) -> (element #1=w593:dbl[], element #2=w592:dbl[])  [unwired: 3 in]
              n365 = local read "x'"() -> (w595:dbl)
              n366 = local read "y'"() -> (w594:dbl)
              n367 = Subtract(x=w593, y=w595) -> (x-y=w591:dbl[])
              n368 = Subtract(x=w592, y=w594) -> (x-y=w590:dbl[])
              n369 = local read "R'"() -> (w599:dbl[][])
              n370 = Build Array(w591, w590) -> (w589:dbl[][])
              n371 = Transpose 2D Array(2D array=w599) -> (transposed array=w598:dbl[][])
              n372 = call-poly <vilib>:"A x B.vi"("B"=w589, "A"=w598) -> ("A x B"=w602:T3)  [unwired: 1 out]
              n373 = Index Array(array=w602, index (row) #1=0 ("index (row)")) -> (element #1=w588:dbl[], element #2=w587:dbl[])  [unwired: 3 in]
              n374 = Build Array(w588, w587) -> (w601:dbl[][])
              n375 = Transpose 2D Array(2D array=w601) -> (transposed array=w585:dbl[][])
              n376 = flat-sequence {
                tunnel: w585 -> [w605]
                tunnel: [w604] -> w584
                frame #0 {
                  n377 = Index Array(array=w605, index (col) #1=0 ("disabled index (col)")) -> (element #1=w626:dbl[], element #2=w621:dbl[])  [unwired: 3 in]
                  n378 = In Range and Coerce(upper limit=40.0, x=w621, lower limit=0.0) -> (In Range?=w619:bool[])  [unwired: 1 out]
                  n379 = In Range and Coerce(upper limit=40.0, x=w626, lower limit=-40.0) -> (In Range?=w620:bool[])  [unwired: 1 out]
                  n380 = Compound Arithmetic op=AND(w620, w619) -> (w606:bool[])
                  n381 = Index Array(array=w605, index (col) #1=0 ("disabled index (col)")) -> (element #1=w608:dbl[], element #2=w607:dbl[])  [unwired: 5 in, 1 out]
                  n382 = Boolean To (0,1)(Boolean=w606) -> (0, 1=w614:i16[])
                  n383 = Build Cluster Array(w606, w608, w607) -> (w612:T4)
                  n384 = To Long Integer(number=w614) -> (32bit integer=w615:i32[])
                  n385 = Sort 1D Array(array=w612) -> (sorted array=w613:T4)
                  n386 = Add Array Elements(numeric array=w615) -> (sum=w616:i32)
                  n387 = Reverse 1D Array(array=w613) -> (reversed array=w617:T4)
                  n388 = for {
                    N: w616 -> [_]
                    tunnel: w617 -> [w630] mode=indexing
                    tunnel: [w629] -> w611 mode=indexing
                    tunnel: [w628] -> w610 mode=indexing
                    n389 = Unbundle(w630) -> ("Real Matrix Element"=w629:dbl, "Real Matrix Element"=w628:dbl)  [unwired: 1 out]
                  }
                  n390 = Build Array(w611, w610) -> (w618:dbl[][])
                  n391 = Transpose 2D Array(2D array=w618) -> (transposed array=w604:dbl[][])
                }
              }
              n392 = local read "mindata"() -> (w586:dbl[][])
              n393 = Build Array (concatenate)(w586, w584) -> (w600:dbl[][])
              n394 = global write "G_SEN.vi" "mindata"(w600) -> ()
            }
            frame Disabled {
              n395 = local read "mindata"() -> (w631:dbl[][])
              n396 = global write "G_SEN.vi" "mindata"(w631) -> ()
            }
          }
          n397 = local read "keydata"() -> (w582:dbl[][])
          n398 = global write "G_SEN.vi" "pos_velo_key"(w583) -> ()
          n399 = global write "G_SEN.vi" "keydata"(w582) -> ()
        }
      }
    }
  }
